vi "Apply_Destination_Edit.vi"(8 "error in (no error)":errorcluster, 10 "edit":T1, 11 "IB_Tree_Dest in":refnum<class "IB_Tree_Dest.lvclass">) -> (0 "error out":errorcluster, 3 "IB_Tree_Dest out":refnum<class "IB_Tree_Dest.lvclass">)   [LabVIEW 2020, in "IB_Tree_Dest.lvclass"]
uses:
  <vilib>/AppBuilder/IB_Classes/Tree_Dest/IB_Tree_Dest.lvclass
  <vilib>/AppBuilder/IB_Classes/Tree_Dest/IB_Tree_Dest.lvclass/IB_Tree_Dest.ctl
  <vilib>/AppBuilder/IB_Classes/Tree/IB_Tree.lvclass
  <vilib>/AppBuilder/IB_Classes/Tree_Dest/destEdits_add.ctl
  <vilib>/AppBuilder/IB_Classes/Tree_Dest/destEdits_remove.ctl
  <vilib>/AppBuilder/IB_Classes/Tree_Dest/destEdits_rename.ctl
  <vilib>/AppBuilder/IB_Classes/Tree_Dest/destEdits_sort.ctl
  <vilib>/AppBuilder/IB_Classes/Tree_Dest/destEdits_defaultDirChange.ctl
  e:/builds/penguin/labview/branches/2020/dev/dist/vi.lib/AppBuilder/IB_Classes/Tree/IB_Tree.lvclass
  e:/builds/penguin/labview/branches/2020/dev/dist/vi.lib/AppBuilder/IB_Classes/Tree_Dest/IB_Tree_Dest.lvclass
  <vilib>/AppBuilder/IB_Classes/Tree_Dest/destEdits_operation.ctl
  <vilib>/AppBuilder/IB_Classes/Tree_Dest/destEdits_edit.ctl
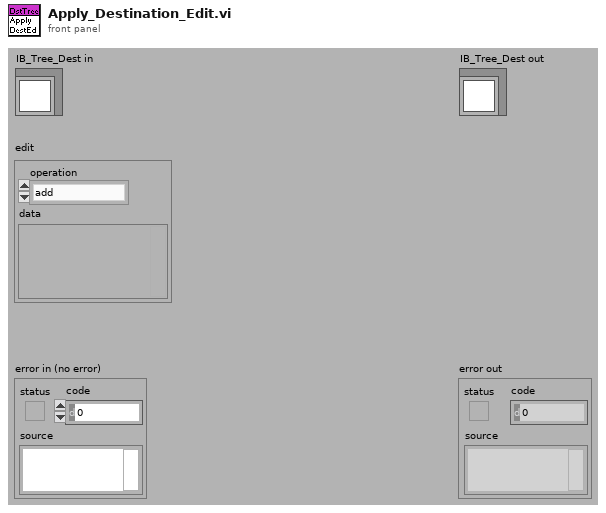
[diagram p1: front panel]
types:
  T1 = typedef "destEdits_edit.ctl" = cluster{"operation":T2, "data":variant}
  T2 = typedef "destEdits_operation.ctl" = enum16{"add", "remove", "rename", "sort children", "default dir changed"}
  T3 = typedef "destEdits_add.ctl" = cluster{"parent tag":string, "child tag":string, "left cell string":string, "symbol index":i32}
  T4 = typedef "destEdits_remove.ctl" = cluster{"child tag":string}
  T5 = typedef "destEdits_sort.ctl" = cluster{"parent tag":string}
  T6 = typedef "destEdits_rename.ctl" = cluster{"child tag":string, "left cell string":string}
  T7 = typedef "destEdits_defaultDirChange.ctl" = cluster{"old default":string, "new default":string}
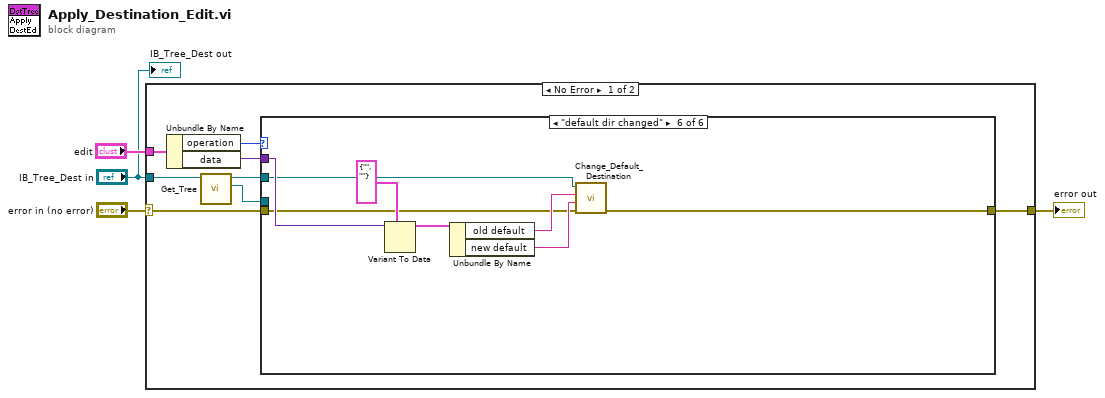
[diagram p0: block diagram]
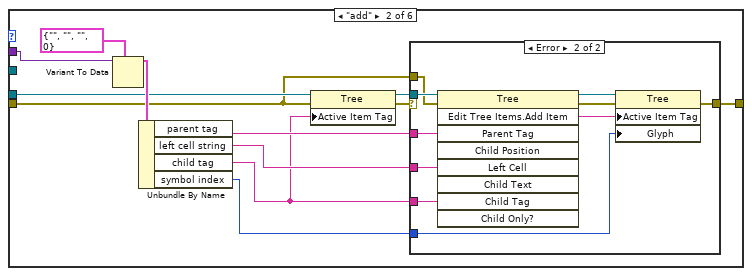
[diagram p3: hidden frame]
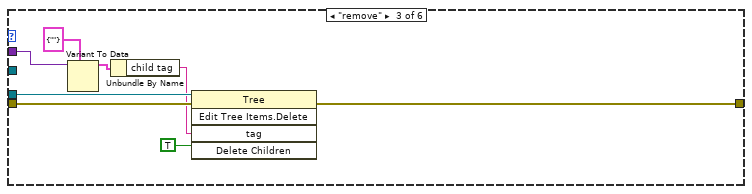
[diagram p5: hidden frame]
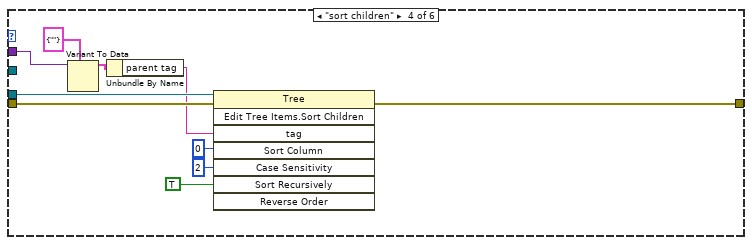
[diagram p6: hidden frame]
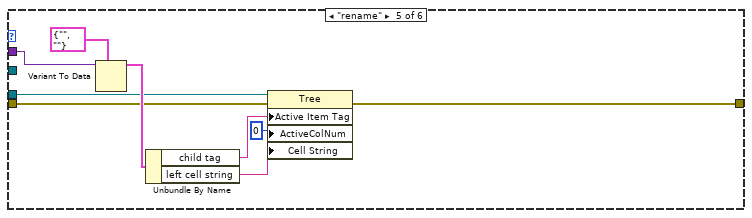
[diagram p7: hidden frame]
diagram:
  n1 = case shown="No Error" "error in (no error)" {
    selector: "error in (no error)" -> [w10 w72]
    tunnel: [w9 w72] -> w2
    tunnel: "IB_Tree_Dest in" -> [w11 _]
    tunnel: "edit" -> [w6 _]
    frame No Error {
      n2 = Unbundle By Name(w6) -> ("operation"=w8:T2, "data"=w7:variant)
      n3 = call <vilib>:"Get_Tree.vi"("IB_Tree in"=w11) -> ("ctl"=w12:refnum<vi>, "IB_Tree out"=w5:refnum<class "IB_Tree_Dest.lvclass">)  [unwired: 1 in, 8 out]
      n4 = case shown="\"default dir changed\"" w8 {
        tunnel: w7 -> [_ w25 w43 w53 w62 w70]
        tunnel: w12 -> [_ w18 w42 w52 w58 _]
        tunnel: w10 -> [w13 w14 w40 w50 w60 w65]
        tunnel: [w13 w20 w39 w49 w59 w64] -> w9
        tunnel: w5 -> [_ _ _ _ _ w68]
        frame Default {
        }
        frame "add" {
          n5 = Variant To Data(type=T3 {"parent tag"="", "child tag"="", "left cell string"="", "symbol index"=0} ("add"), Variant=w25) -> (data=w23:T3)  [unwired: 1 in, 1 out]
          n6 = Unbundle By Name(w23) -> ("parent tag"=w22:string, "left cell string"=w21:string, "child tag"=w16:string, "symbol index"=w19:i32)
          n7 = property class="Tree"(reference=w18, error in=w14, "Active Item Tag"=w16) -> (reference out=w17:refnum<vi>, error out=w15:errorcluster)
          n8 = case shown="Error" w15 {
            selector: w15 -> [w26 _]
            tunnel: w22 -> [_ w36]
            tunnel: w21 -> [_ w35]
            tunnel: [w26 w31] -> w20
            tunnel: w19 -> [_ w30]
            tunnel: w17 -> [_ w29]
            tunnel: w16 -> [_ w28]
            tunnel: w14 -> [_ w27]
            frame No Error {
              # "do not add if already present"
            }
            frame Error {
              n9 = invoke class="Tree" method="Edit Tree Items.Add Item"(reference=w29, error in=w27, "Parent Tag"=w36, "Left Cell"=w35, "Child Tag"=w28) -> (reference out=w34:refnum<vi>, error out=w32:errorcluster, "Edit Tree Items:Add Item"=w33:string)  [unwired: 4 in, 6 out]
              n10 = property class="Tree"(reference=w34, error in=w32, "Active Item Tag"=w33, "Glyph"=w30) -> (error out=w31:errorcluster)  [unwired: 1 out]
            }
          }
        }
        frame "remove" {
          n11 = Variant To Data(type=T4 {"child tag"=""} ("remove"), Variant=w43) -> (data=w41:T4)  [unwired: 1 in, 1 out]
          n12 = Unbundle By Name(w41) -> ("child tag"=w38:string)
          n13 = invoke class="Tree" method="Edit Tree Items.Delete"(reference=w42, error in=w40, "tag"=w38, "Delete Children"=TRUE ("Delete Children?")) -> (error out=w39:errorcluster)  [unwired: 1 in, 4 out]
        }
        frame "sort children" {
          n14 = Variant To Data(type=T5 {"parent tag"=""} ("sort"), Variant=w53) -> (data=w51:T5)  [unwired: 1 in, 1 out]
          n15 = Unbundle By Name(w51) -> ("parent tag"=w48:string)
          n16 = invoke class="Tree" method="Edit Tree Items.Sort Children"(reference=w52, error in=w50, "tag"=w48, "Sort Column"=0, "Case Sensitivity"=2, "Sort Recursively"=TRUE ("Delete Children?")) -> (error out=w49:errorcluster)  [unwired: 2 in, 7 out]
        }
        frame "rename" {
          n17 = Variant To Data(type=T6 {"child tag"="", "left cell string"=""} ("rename"), Variant=w62) -> (data=w61:T6)  [unwired: 1 in, 1 out]
          n18 = Unbundle By Name(w61) -> ("child tag"=w57:string, "left cell string"=w55:string)
          n19 = property class="Tree"(reference=w58, error in=w60, "Active Item Tag"=w57, "ActiveColNum"=0 ("Active Cell:Active Column Number"), "Cell String"=w55) -> (error out=w59:errorcluster)  [unwired: 1 out]
        }
        frame "default dir changed" {
          n20 = Variant To Data(type=T7 {"old default"="", "new default"=""} ("remove"), Variant=w70) -> (data=w69:T7)  [unwired: 1 in, 1 out]
          n21 = Unbundle By Name(w69) -> ("old default"=w67:string, "new default"=w66:string)
          n22 = call <vilib>:"Change_Default_Destination.vi"("error in (no error)"=w65, "New default dest"=w66, "Old default dest"=w67, "IB_DestTree in"=w68) -> ("error out"=w64:errorcluster)  [unwired: 7 out]
        }
      }
    }
    frame Error {
    }
  }
  "error out" <- w2
  "IB_Tree_Dest out" <- "IB_Tree_Dest in"
